vi "Process Sequence Triggers.vi"() -> ()   [LabVIEW 2015]
uses:
  Sequence Global Action.ctl
  Sensors/Sensor Data Global Action.ctl
  Sequence File IO/Test Sequence Trigger.ctl
  Sensors/Sensor Enum.ctl
panel:
  in  "Last Sequence Time":i32
  in  "Current Sequence Time":i32
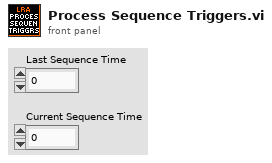
[diagram p1: front panel]
types:
  T1 = typedef "Sensor Data Global Action.ctl" = enum16{"Get Data", "Decode & Store Data"}
  T2 = typedef "Sequence Global Action.ctl" = enum16{"Get", "Set List", "Set Current"}
  T3 = typedef "Single Test Sequence.ctl" = cluster{"Actions":T4[], "Triggers":T7[], "Name":string}
  T4 = typedef "Test Sequence Action.ctl" = cluster{"Time":i32, "Action":T5, "Valve":T6}
  T5 = typedef "Valve Action Enum.ctl" = enum16{"Open", "Close"}
  T6 = typedef "Valve Name Enum.ctl" = enum16{"FV-2", "FV-3", "FV-4", "OV-2", "OV-3", "OV-4", "COMP"}
  T7 = typedef "Test Sequence Trigger.ctl" = cluster{"Sensor":T8, "Begin Time (ms)":u32, "End Time(ms)":u32, "Min Value":dbl, "Max Value":dbl, "Exceed Action":string}
  T8 = typedef "Sensor Enum.ctl" = enum16{"FPD-1", "FPD-2", "FPD-3", "OPD-1", "OPD-2", "OPD-3", "AP-1", "VBAT", "VCOMP", "ICOMP", "TD10"}
  T9 = typedef "Transducer Calibration Display.ctl" = cluster{"Value":dbl, "Raw":dbl, "Scaled":dbl, "Sensor Name":T8, "Port":u32}
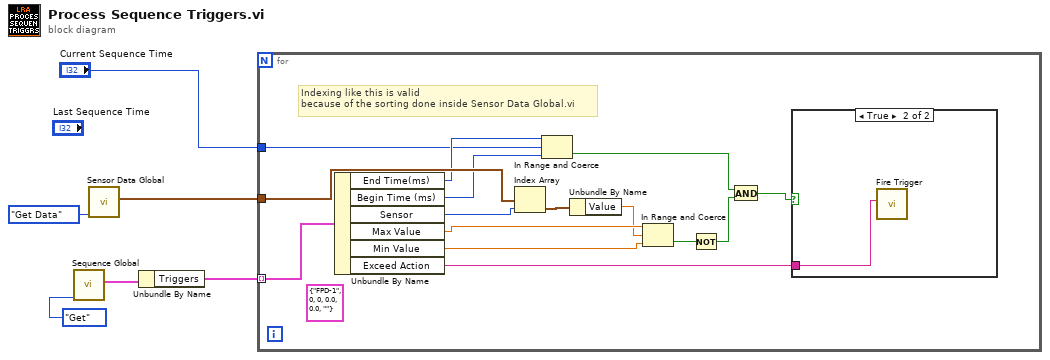
[diagram p0: block diagram]
diagram:
  n1 = call "Sequence Global.vi"("Action"=Sequence_Global_Action."Get") -> ("Current Sequence"=w6:T3)  [unwired: 8 in, 2 out]
  n2 = call "Sensor Data Global.vi"("Command"=Sensor_Data_Global_Action."Get Data") -> ("Sensor Data"=w2:T9[])  [unwired: 10 in]
  n3 = Unbundle By Name(w6) -> ("Triggers"=w4:T7[])
  n4 = for {
    tunnel: w4 -> [w21] mode=indexing
    tunnel: w2 -> [w20]
    tunnel: "Current Sequence Time" -> [w12]
    (unwired) T7 {"Sensor"=enum."FPD-1", "Begin Time (ms)"=0, "End Time(ms)"=0, "Min Value"=0.0, "Max Value"=0.0, "Exceed Action"=""}
    # "Indexing like this is valid\nbecause of the sorting done inside Sensor Data Global.vi"
    n5 = Unbundle By Name(w21) -> ("End Time(ms)"=w13:u32, "Begin Time (ms)"=w14:u32, "Sensor"=w15:T8, "Max Value"=w18:dbl, "Min Value"=w17:dbl, "Exceed Action"=w7:string)
    n6 = Index Array(array=w20, index=w15) -> (element=w19:T9)
    n7 = In Range and Coerce(upper limit=w13, x=w12, lower limit=w14) -> (In Range?=w9:bool)  [unwired: 1 out]
    n8 = Unbundle By Name(w19) -> ("Value"=w16:dbl)
    n9 = In Range and Coerce(upper limit=w18, x=w16, lower limit=w17) -> (In Range?=w11:bool)  [unwired: 1 out]
    n10 = Not(x=w11) -> (.not. x?=w10:bool)
    n11 = And(x=w9, y=w10) -> (x .and. y?=w8:bool)
    n12 = case shown="True" w8 {
      tunnel: w7 -> [_ w22]
      frame False {
      }
      frame True {
        n13 = call "Fire Trigger.vi"("Exceed Action"=w22) -> ()  [unwired: 11 in]
      }
    }
  }
